vi "Static Write.vi"(8 "error in (no error)":errorcluster, 10 "Value":i8, 11 "Abs_I8 Integer in":refnum<class "Abs_I8 Integer.lvclass">) -> (0 "error out":errorcluster, 3 "Abs_I8 Integer out":refnum<class "Abs_I8 Integer.lvclass">)   [LabVIEW 2021, in "Abs_I8 Integer.lvclass"]
uses:
  Abs_I8 Integer.lvclass
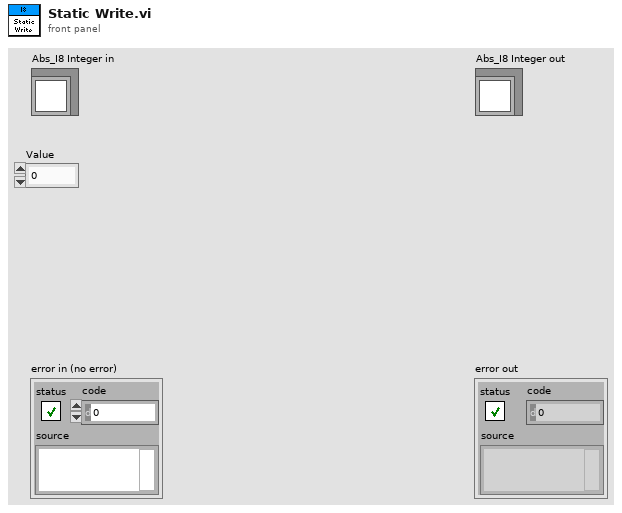
[diagram p1: front panel]
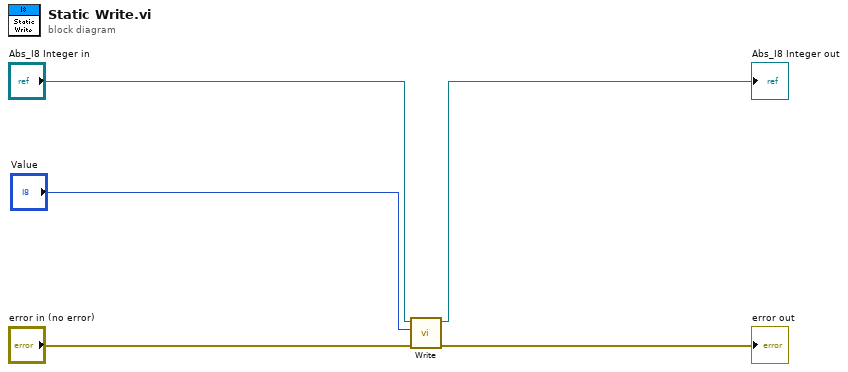
[diagram p0: block diagram]
diagram:
  n1 = call-dynamic "Write.vi"("error in (no error)"="error in (no error)", "Value"="Value", "Double Float.lvclass_340760 in"="Abs_I8 Integer in") -> ("error out"=→"error out":errorcluster, "Double Float.lvclass_340760 out"=→"Abs_I8 Integer out":refnum<class "Abs_I8 Integer.lvclass">)  [unwired: 7 in]
